vi "ADAM_Read.vi"(8 "错误输入（无错误）":errorcluster, 11 "VISA resource name":refnum<visa-resource-name> caption="VISA资源名称") -> (0 "error out":errorcluster caption="错误输出", 1 "humidity":dbl, 2 "temperature":dbl, 3 "Data":string)   [LabVIEW 2017]
panel:
  out "长度 2":i32
  out "长度":i32
  out "HumidityValue":string
  out "TemperatureValue":string
  in  "Command":string="010300010002\n"
  out "Data 2":T1
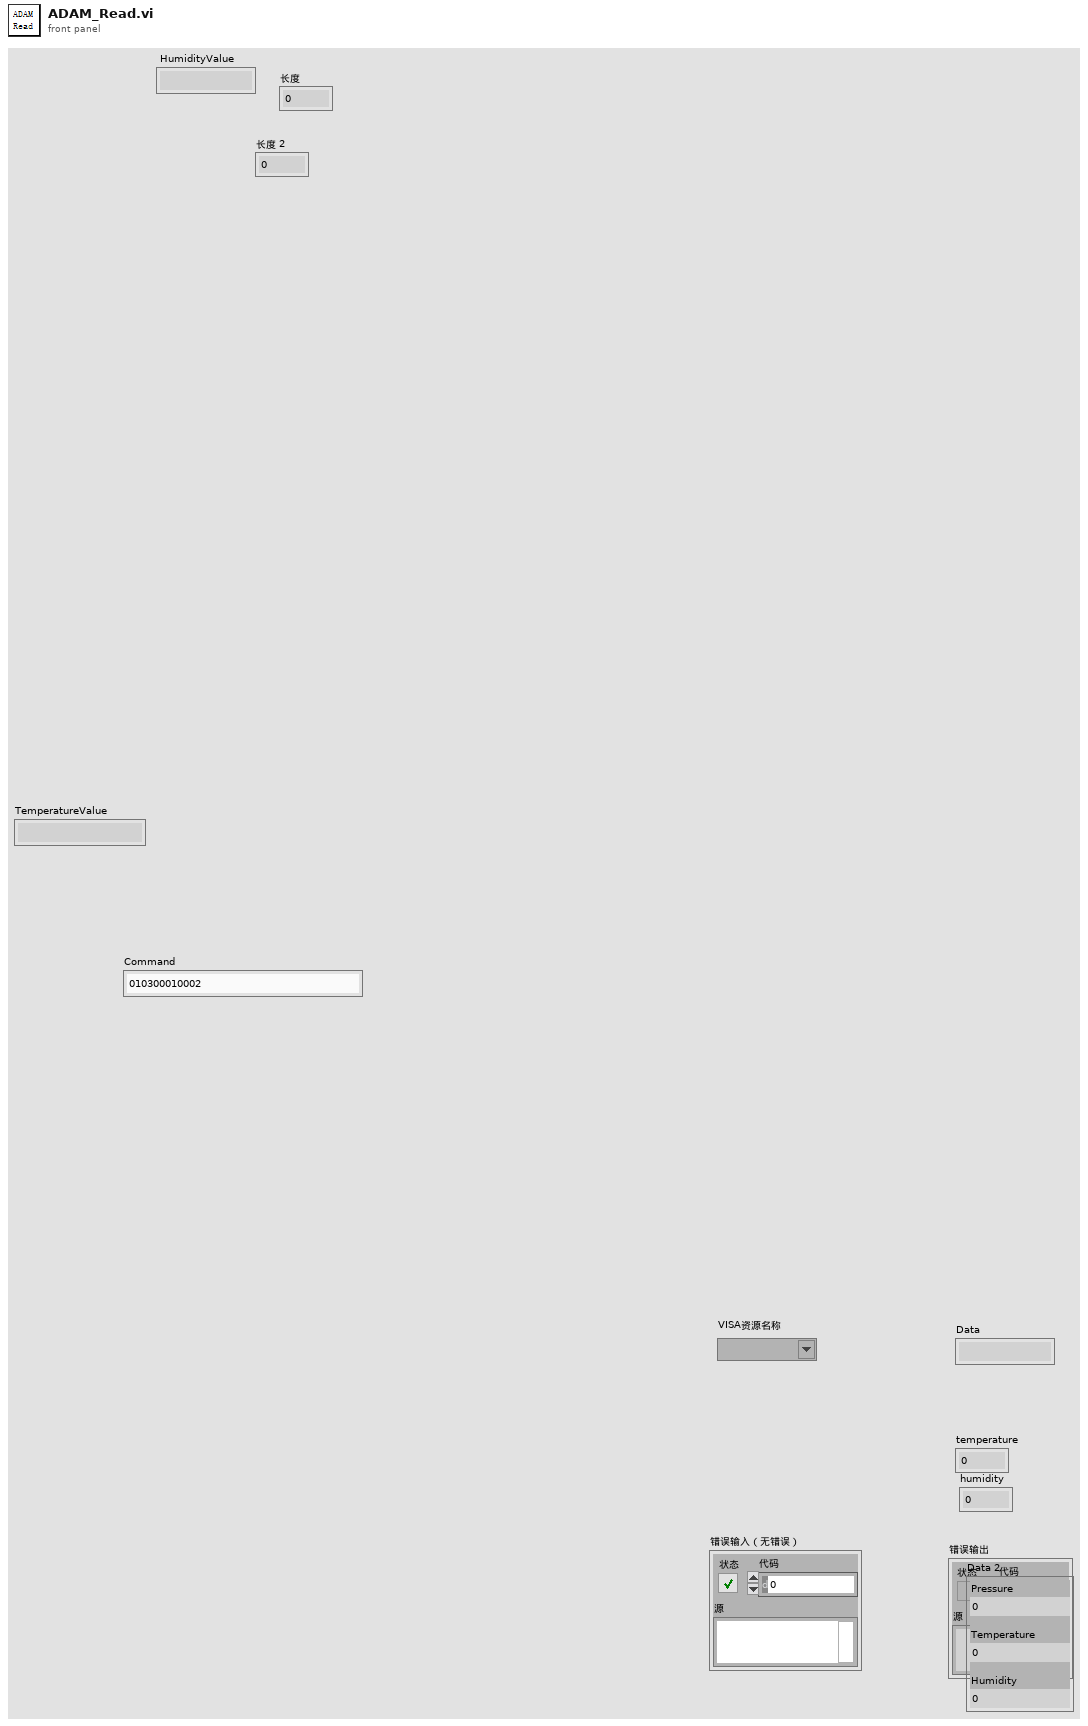
[diagram p1: front panel]
types:
  T1 = cluster{"Pressure":dbl, "Temperature":dbl, "Humidity":dbl}
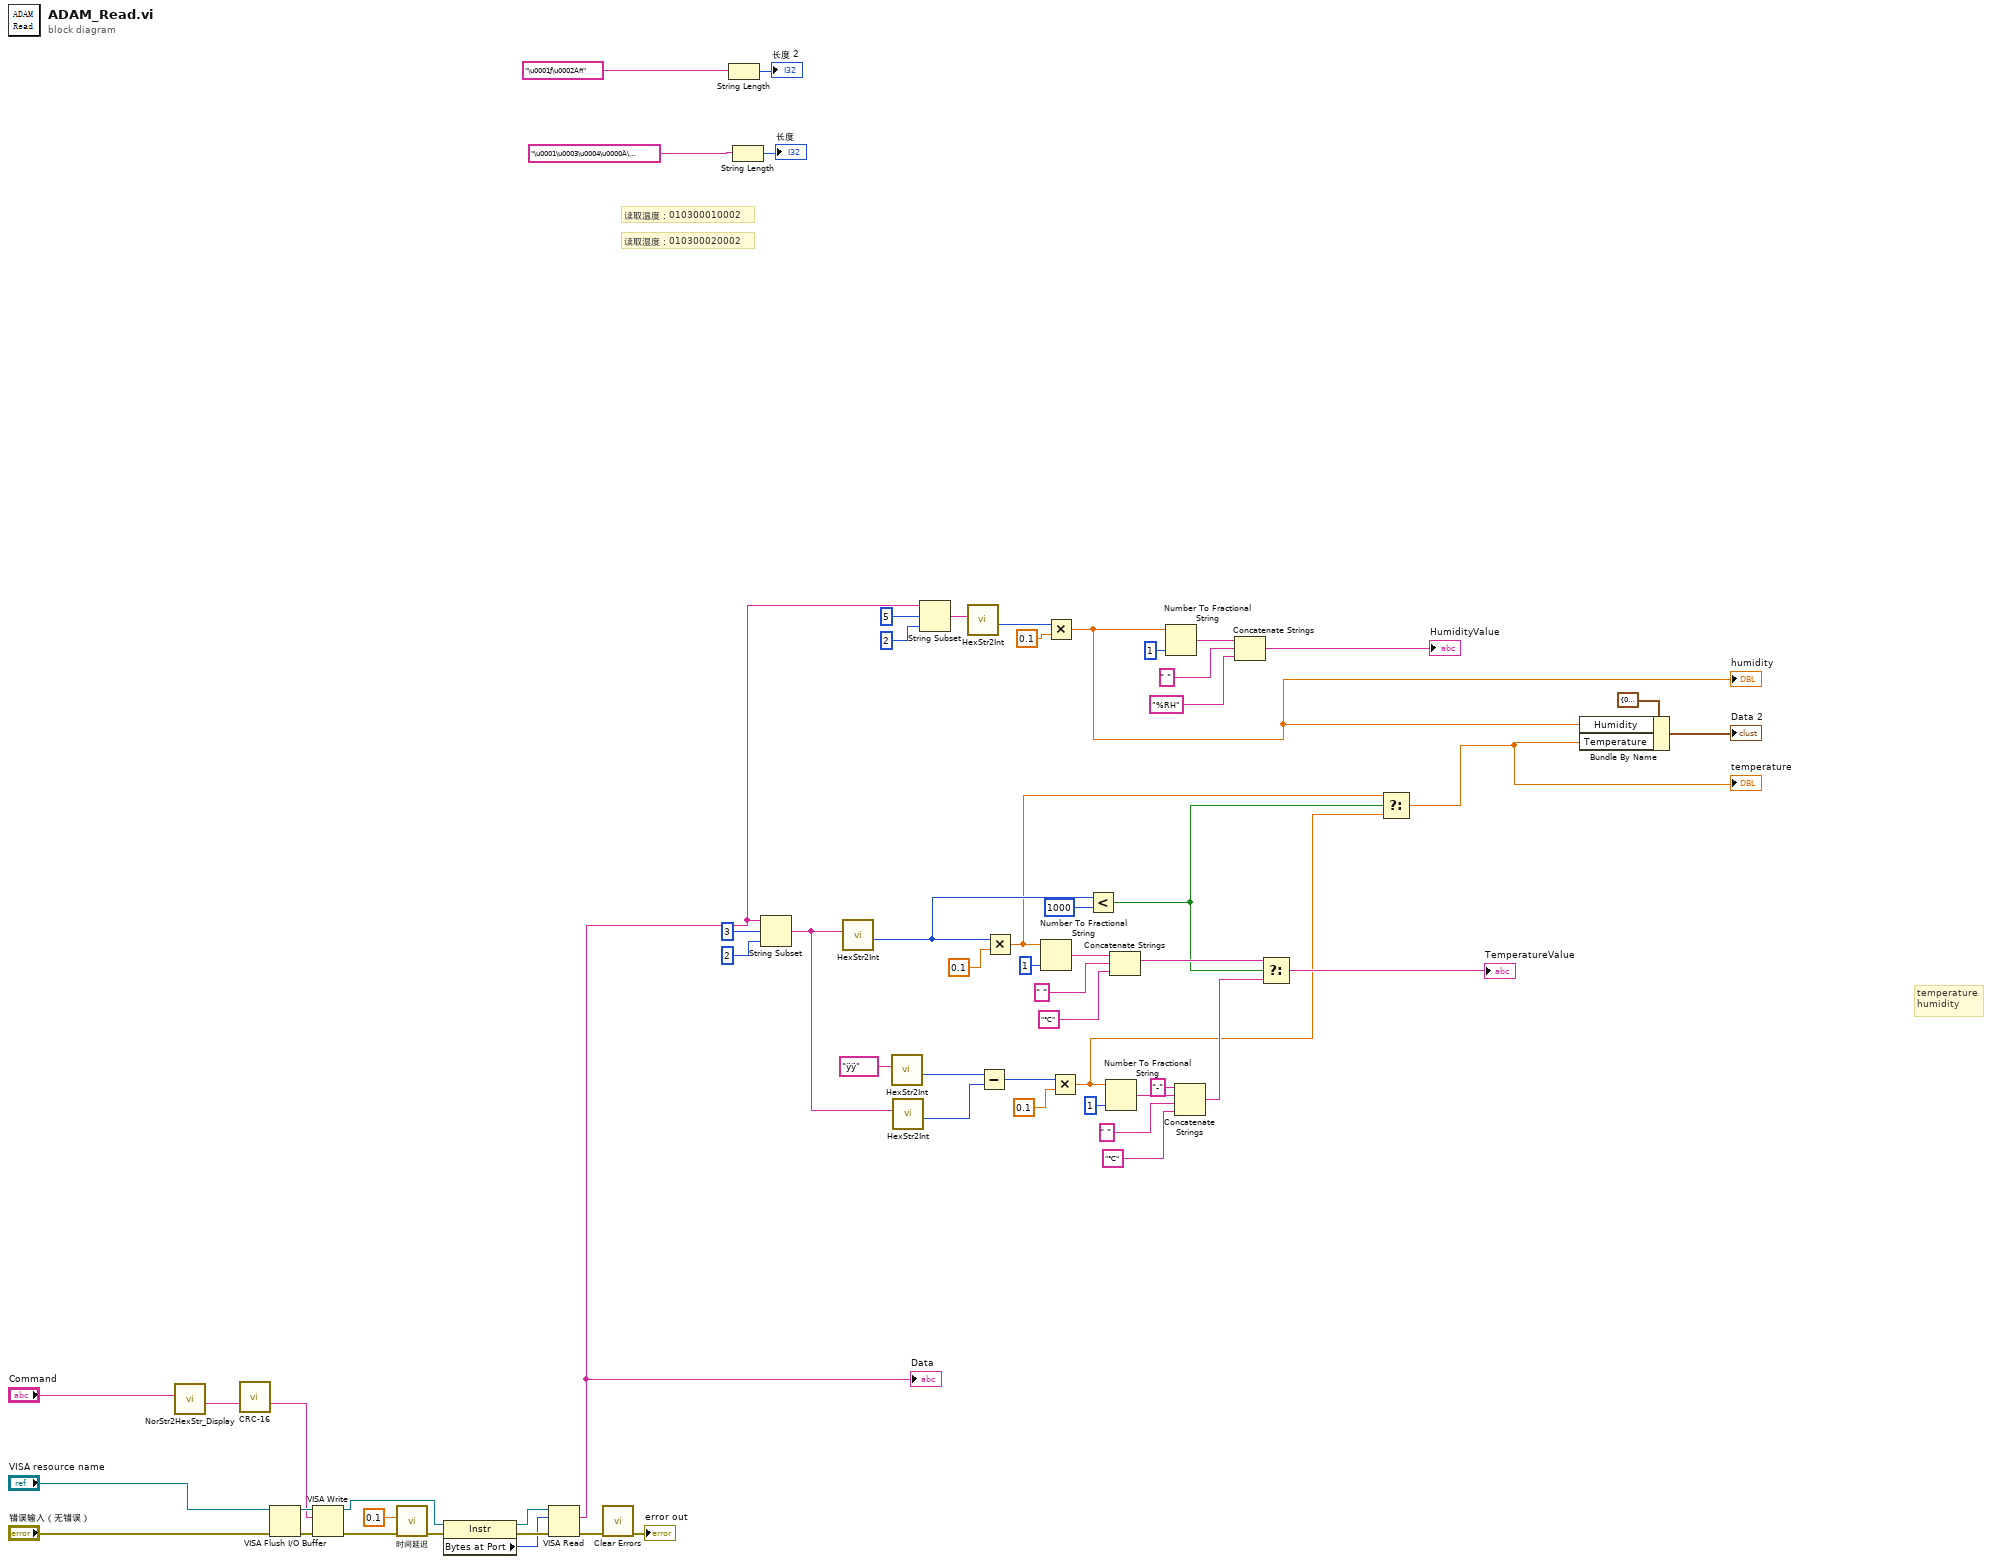
[diagram p0: block diagram]
diagram:
  # "读取湿度：010300020002"
  # "读取温度：010300010002"
  # "temperature\nhumidity"
  n1 = call "NorStr2HexStr_Display.vi"("Normal Display"="Command") -> ("Hex Display"=w46:string)  [unwired: 10 in]
  n2 = call "CRC-16.vi"("string_hex"=w46) -> ("string&CRC-16"=w7:string)  [unwired: 14 in]
  n3 = VISA Flush I/O Buffer(VISA resource name="VISA resource name", error in (no error)="错误输入（无错误）") -> (VISA resource name out=w61:refnum<visa-resource-name>, error out=w59:errorcluster)  [unwired: 1 in]
  n4 = VISA Write(VISA resource name=w61, write buffer=w7, error in (no error)=w59) -> (VISA resource name out=w53:refnum<visa-resource-name>, error out=w60:errorcluster)  [unwired: 1 out]
  n5 = call "时间延迟"("error in (no error)"=w60, "Delay Time (s)"=0.1) -> ("error out"=w50:errorcluster)  [unwired: 9 in]
  n6 = property class="Instr"(reference=w53, error in=w50) -> (reference out=w52:refnum<visa-resource-name>, error out=w51:errorcluster, "Bytes at Port"=w49:u32)
  n7 = VISA Read(VISA resource name=w52, byte count=w49, error in (no error)=w51) -> (read buffer=w6:string, error out=w58:errorcluster)  [unwired: 2 out]
  "Data" <- w6
  n8 = call <vilib>:"Clear Errors.vi"("error in (no error)"=w58) -> ("error out"=→"error out":errorcluster)  [unwired: 5 in, 1 out]
  n9 = String Length(string="\u0001ƒ\u0002Àñ" ("字符串")) -> (length=→"长度 2":i32)
  n10 = String Length(string="\u0001\u0003\u0004\u0000Ä\u00014»‰" ("字符串")) -> (length=→"长度":i32)
  n11 = String Subset(string=w6, offset (0)=3 ("偏移量(0)"), length (rest)=2 ("长度（剩余）")) -> (substring=w23:string)
  n12 = call "HexStr2Int.vi"("十六进制字符串"=w23) -> ("数字"=w24:u32)  [unwired: 10 in]
  n13 = call "HexStr2Int.vi"("十六进制字符串"="ÿÿ") -> ("数字"=w36:u32)  [unwired: 10 in]
  n14 = call "HexStr2Int.vi"("十六进制字符串"=w23) -> ("数字"=w35:u32)  [unwired: 10 in]
  n15 = String Subset(string=w6, offset (0)=5 ("偏移量(0)"), length (rest)=2 ("长度（剩余）")) -> (substring=w22:string)
  n16 = call "HexStr2Int.vi"("十六进制字符串"=w22) -> ("数字"=w21:u32)  [unwired: 10 in]
  n17 = Subtract(x=w36, y=w35) -> (x-y=w29:u32)
  n18 = Multiply(x=w24, y=0.1) -> (x*y=w3:dbl)
  n19 = Number To Fractional String(number=w3, precision (6)=i16 1 ("精度(6)")) -> (F-format string=w38:string)  [unwired: 2 in]
  n20 = Multiply(x=w21, y=0.1) -> (x*y=w2:dbl)
  "humidity" <- w2
  n21 = Multiply(x=w29, y=0.1) -> (x*y=w4:dbl)
  n22 = Less?(x=w24, y=u32 1000) -> (x < y?=w5:bool)
  n23 = Number To Fractional String(number=w4, precision (6)=i16 1 ("精度(6)")) -> (F-format string=w34:string)  [unwired: 2 in]
  n24 = Concatenate Strings(w38, " " ("字符串"), "℃" ("字符串")) -> (w26:string)
  n25 = Number To Fractional String(number=w2, precision (6)=i16 1 ("精度(6)")) -> (F-format string=w20:string)  [unwired: 2 in]
  n26 = Concatenate Strings("-" ("字符串"), w34, " " ("字符串"), "℃" ("字符串")) -> (w25:string)
  n27 = Concatenate Strings(w20, " " ("字符串"), "%RH" ("字符串")) -> (→"HumidityValue":string)
  n28 = Select(t=w26, s=w5, f=w25) -> (s? t:f=→"TemperatureValue":string)
  n29 = Select(t=w3, s=w5, f=w4) -> (s? t:f=w1:dbl)
  "temperature" <- w1
  n30 = Bundle By Name(cluster=T1 {"Pressure"=0.0, "Temperature"=0.0, "Humidity"=0.0} ("Data"), "Humidity"=w2, "Temperature"=w1) -> (→"Data 2":T1)
